vi "Graph Save Scale(Mixed).vi"(8 "err in":errorcluster caption="エラー入力（エラーなし）", 11 "MixedGraph入力":refnum<vi>) -> (0 "error out":errorcluster caption="エラー出力")   [LabVIEW 2014]
uses:
  TypeDef/PlotParam.ctl
  TypeDef/ScaleParam.ctl
  <vilib>/Utility/miscctls.llb/LVRangeTypeDef.ctl
  <vilib>/Utility/xml.llb/Write to XML File(string).vi
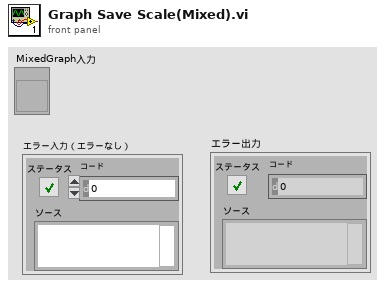
[diagram p1: front panel]
types:
  T1 = typedef "ScaleParam.ctl" = cluster{"NameLbl.Text":string, "UnitLabel.Text":string, "Range":T2}
  T2 = typedef "LVRangeTypeDef.ctl" = cluster{"Minimum":dbl, "Maximum":dbl, "Increment":dbl, "Minor Increment":dbl, "Start":dbl}
  T3 = typedef "PlotParam.ctl" = cluster{"Plot Color":u32, "Point Style":u8, "Line Width":u8, "Visible?":bool, "XScaleIdx":u32, "YScaleIdx":u32}
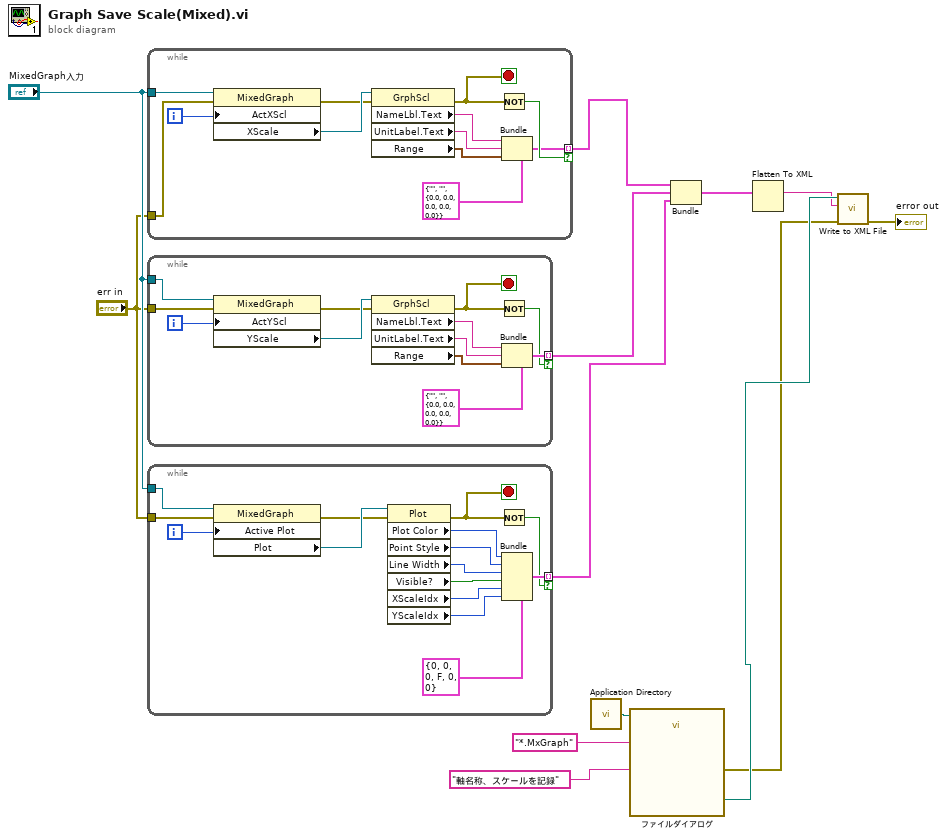
[diagram p0: block diagram]
diagram:
  n1 = while {
    tunnel: "err in" -> [w25]
    tunnel: "MixedGraph入力" -> [w23]
    tunnel: [w14] -> w8 mode=indexing if=w17
    i -> [w19]
    stop <- w16 stop-if-true
    n2 = property class="MixedGraph"(reference=w23, error in=w25, "ActXScl"=w19) -> (error out=w18:errorcluster, "XScale"=w24:refnum<vi>)  [unwired: 1 out]
    n3 = property class="GrphScl"(reference=w24, error in=w18) -> (error out=w16:errorcluster, "NameLbl.Text"=w22:string, "UnitLabel.Text"=w21:string, "Range"=w20:T2)  [unwired: 1 out]
    n4 = Not(x=w16) -> (.not. x?=w17:bool)
    n5 = Bundle(cluster=T1 {"NameLbl.Text"="", "UnitLabel.Text"="", "Range"={"Minimum"=0.0, "Maximum"=0.0, "Increment"=0.0, "Minor Increment"=0.0, "Start"=0.0}} ("出力クラスタ"), "NameLbl.Text"=w22, "UnitLabel.Text"=w21, "Range"=w20) -> (w14:T1)
  }
  n6 = while {
    tunnel: "err in" -> [w37]
    tunnel: "MixedGraph入力" -> [w35]
    tunnel: [w31] -> w7 mode=indexing if=w28
    i -> [w30]
    stop <- w27 stop-if-true
    n7 = property class="MixedGraph"(reference=w35, error in=w37, "ActYScl"=w30) -> (error out=w29:errorcluster, "YScale"=w36:refnum<vi>)  [unwired: 1 out]
    n8 = property class="GrphScl"(reference=w36, error in=w29) -> (error out=w27:errorcluster, "NameLbl.Text"=w34:string, "UnitLabel.Text"=w33:string, "Range"=w32:T2)  [unwired: 1 out]
    n9 = Not(x=w27) -> (.not. x?=w28:bool)
    n10 = Bundle(cluster=T1 {"NameLbl.Text"="", "UnitLabel.Text"="", "Range"={"Minimum"=0.0, "Maximum"=0.0, "Increment"=0.0, "Minor Increment"=0.0, "Start"=0.0}} ("出力クラスタ"), "NameLbl.Text"=w34, "UnitLabel.Text"=w33, "Range"=w32) -> (w31:T1)
  }
  n11 = while {
    tunnel: "MixedGraph入力" -> [w52]
    tunnel: [w43] -> w6 mode=indexing if=w41
    tunnel: "err in" -> [w39]
    i -> [w51]
    stop <- w42 stop-if-true
    n12 = property class="MixedGraph"(reference=w52, error in=w39, "Active Plot"=w51) -> (error out=w38:errorcluster, "Plot"=w50:refnum<vi>)  [unwired: 1 out]
    n13 = property class="Plot"(reference=w50, error in=w38) -> (error out=w42:errorcluster, "Plot Color"=w49:u32, "Point Style"=w48:u8, "Line Width"=w47:u8, "Visible?"=w46:bool, "XScaleIdx"=w45:u32, "YScaleIdx"=w44:u32)  [unwired: 1 out]
    n14 = Not(x=w42) -> (.not. x?=w41:bool)
    n15 = Bundle(cluster=T3 {"Plot Color"=0, "Point Style"=0, "Line Width"=0, "Visible?"=FALSE, "XScaleIdx"=0, "YScaleIdx"=0} ("出力クラスタ"), "Plot Color"=w49, "Point Style"=w48, "Line Width"=w47, "Visible?"=w46, "XScaleIdx"=w45, "YScaleIdx"=w44) -> (w43:T3)
  }
  n16 = call <vilib>:"Application Directory.vi"() -> ("Application Directory"=w13:path)
  n17 = call "ファイルダイアログ"("start path"=w13, "prompt"="軸名称、スケールを記録", "pattern (all files)"="*.MxGraph") -> ("selected path"=w5:path, "error out"=w2:errorcluster)  [unwired: 9 in, 2 out]
  n18 = Bundle(w8, w7, w6) -> (w4:cluster{T1[], T1[], T3[]})  [unwired: 1 in]
  n19 = Flatten To XML(anything=w4) -> (xml string=w3:string)
  n20 = call-poly <vilib>:"Write to XML File.vi"("error in (no error)"=w2, "XML Input"=w3, "XML File Path"=w5) -> ("error out"=→"error out":errorcluster)  [unwired: 6 in, 2 out]
